vi "Particle Analysis Report.vi"() -> ()   [LabVIEW 2014]
doc: "This example introduces the processing area of particle analysis. This example uses the threshold function that converts a grayscale image into a binary image."
uses:
  <vilib>/vision/NI_Vision_Development_Module.lvlib
panel:
  in  "Stop":bool
  out "Selected Particle Report":T1 {"Orientation" format="%.2f"; "Center of Mass"."Y" format="%.2f"; "Center of Mass"."X" format="%.2f"}
  in  "Selected Particle":i32(slide)=2 min=1 max=34 scale=0.0..34.0
  out "Threshold Image":T2(plugin-control)
  # "Overview: Demonstrates how to use the IMAQ Particle Analysis Report function with a binary image to return information about each particle.\nRequirements: Vision Development Software.\nInstructions:\n1. Run the VI.\n2. Change the Selected Particle to update the Selected Particle Report, and overlay the bounding box for the selected particle."
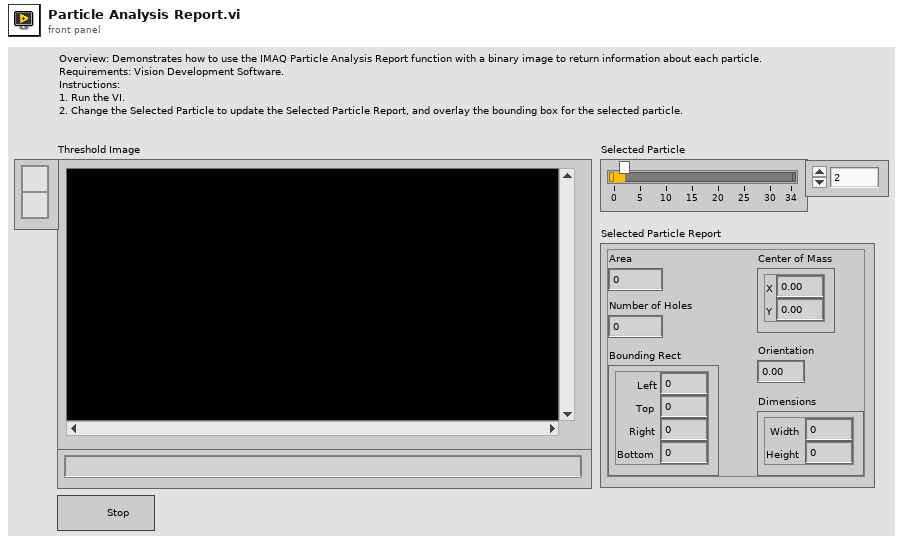
[diagram p1: front panel]
types:
  T1 = cluster{"Area":dbl, "Number of Holes":dbl, "Bounding Rect":cluster{"Left":dbl, "Top":dbl, "Right":dbl, "Bottom":dbl}, "Center of Mass":cluster{"X":dbl, "Y":dbl}, "Orientation":dbl, "Dimensions":cluster{"Width":dbl, "Height":dbl}}
  T2 = typedef "IMAQ Image.ctl" = refnum<image>
  T3 = cluster{"Area":dbl, "Number of Holes":dbl, "Bounding Rect":cluster{"Left":dbl, "Top":dbl, "Right":dbl, "Bottom":dbl}, "Center of Mass":cluster{"X":dbl, "Y":dbl}, "Orientation":dbl, "Dimensions":cluster{"Width":dbl, "Height":dbl}}[]
  T4 = cluster{"Left":dbl, "Top":dbl, "Right":dbl, "Bottom":dbl}
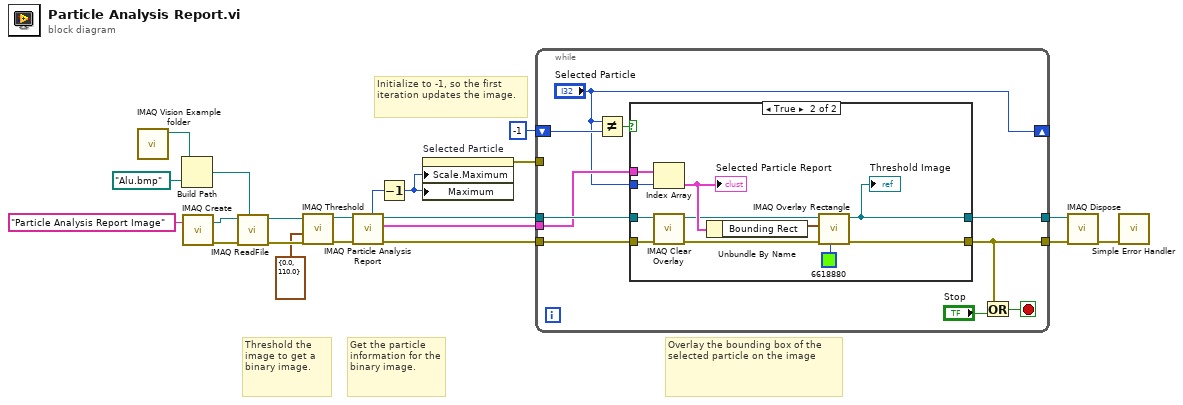
[diagram p0: block diagram]
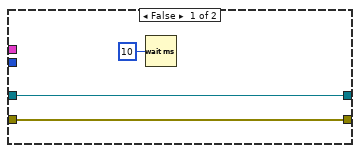
[diagram p2: hidden frame]
diagram:
  # "Initialize to -1, so the first iteration updates the image."
  # "Overlay the bounding box of the selected particle on the image"
  # "Get the particle information for the binary image."
  # "Threshold the image to get a binary image."
  n1 = call "IMAQ Vision Example folder.vi"() -> ("Example Image Path"=w18:path)  [unwired: 11 in]
  n2 = Build Path(base path=w18, name or relative path=path "Alu.bmp") -> (appended path=w16:path)
  n3 = call "IMAQ Create"("Image Name"="Particle Analysis Report Image") -> ("New Image"=w20:T2, "error out"=w19:errorcluster)  [unwired: 4 in]
  n4 = call "IMAQ ReadFile"("File Path"=w16, "error in (no error)"=w19, "Image"=w20) -> ("error out"=w14:errorcluster, "Image Out"=w15:T2)  [unwired: 4 in, 3 out]
  n5 = call "IMAQ Threshold"("error in (no error)"=w14, "Range"=cluster{"Lower value":sgl, "Upper value":sgl} {"Lower value"=0.0, "Upper value"=110.0}, "Image Src"=w15) -> ("error out"=w13:errorcluster, "Image Dst Out"=w12:T2)  [unwired: 7 in]
  n6 = call "IMAQ Particle Analysis Report"("error in (no error)"=w13, "Image"=w12) -> ("error out"=w9:errorcluster, "Particle Reports (Pixels)"=w6:T3, "Image Out (duplicate)"=w10:T2, "Number of Particles"=w7:i32)  [unwired: 4 in, 2 out]
  n7 = Decrement(x=w7) -> (x-1=w3:i32)
  n8 = property on="Selected Particle" class="Slide (strict)"("Scale.Maximum"=w3, "Maximum"=w3) -> (error out=w2:errorcluster)  [unwired: 2 in, 1 out]
  n9 = while {
    tunnel: w10 -> [w31]
    tunnel: w9 -> [w30]
    tunnel: [w24] -> w8
    tunnel: [w29] -> w5
    tunnel: w6 -> [w27]
    shift-right: ["Selected Particle"] -> _
    shift-left: -1 ("Selected Particle") -> [w28]
    tunnel: w2 -> [_]
    stop <- w23 stop-if-true
    n10 = Not Equal?(x="Selected Particle", y=w28) -> (x != y?=w26:bool)
    n11 = case shown="True" w26 {
      tunnel: w31 -> [w34 w40]
      tunnel: w30 -> [w33 w39]
      tunnel: [w33 w45] -> w24
      tunnel: [w34 w36] -> w29
      tunnel: w27 -> [_ w42]
      tunnel: "Selected Particle" -> [_ w35]
      frame False {
        n12 = Wait (ms)(milliseconds to wait=u32 10) -> ()  [unwired: 1 out]
      }
      frame True {
        n13 = Index Array(array=w42, index=w35) -> (element=w41:T1)
        "Selected Particle Report" <- w41
        n14 = call "IMAQ Clear Overlay"("error in (no error)"=w39, "Image"=w40) -> ("error out"=w37:errorcluster, "Image Out"=w38:T2)  [unwired: 8 in]
        n15 = Unbundle By Name(w41) -> ("Bounding Rect"=w44:T4)
        n16 = call "IMAQ Overlay Rectangle"("Color"=u32 6618880, "error in (no error)"=w37, "Rectangle"=w44, "Image"=w38) -> ("error out"=w45:errorcluster, "Image Out"=w36:T2)  [unwired: 6 in]
        "Threshold Image" <- w36
      }
    }
    n17 = Or(x=w24, y="Stop") -> (x .or. y?=w23:bool)
  }
  n18 = call "IMAQ Dispose"("Image"=w5, "error in (no error)"=w8) -> ("error out"=w11:errorcluster)  [unwired: 4 in]
  n19 = call <vilib>:"Simple Error Handler.vi"("error in (no error)"=w11) -> ()  [unwired: 4 in, 5 out]
